vi "get_number_hot_cold_pixels.vi"(8 "error in (no error)":errorcluster, 11 "ColorOverlay in":refnum<class "ColorOverlay.lvclass">) -> (0 "error out":errorcluster, 1 "# hot pixels":i32, 2 "# cold pixels":i32, 3 "ColorOverlay out":refnum<class "ColorOverlay.lvclass">)   [LabVIEW 2010, in "ColorOverlay.lvclass"]
uses:
  ColorOverlay.lvclass
  ColorOverlay.lvclass/ColorOverlay.ctl
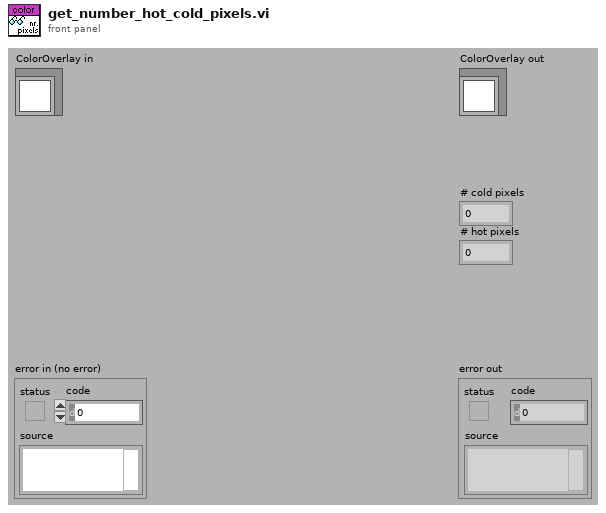
[diagram p1: front panel]
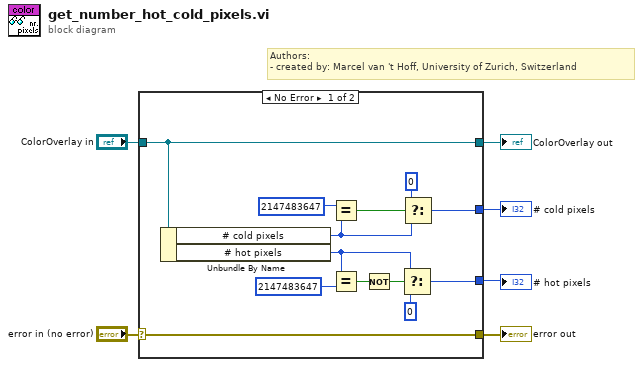
[diagram p0: block diagram]
diagram:
  # "Authors: \n- created by: Marcel van 't Hoff, University of Zurich, Switzerland"
  n1 = case shown="No Error" "error in (no error)" {
    selector: "error in (no error)" -> [w19 w21]
    tunnel: [w19 w21] -> w5
    tunnel: [w18 w20] -> w3
    tunnel: "ColorOverlay in" -> [w18 w20]
    tunnel: [w14 _] -> w2
    tunnel: [w7 _] -> w1
    frame No Error {
      n2 = Unbundle By Name(w18) -> ("# cold pixels"=w15:i32, "# hot pixels"=w8:i32)
      n3 = Equal?(x=2147483647, y=w15) -> (x = y?=w16:bool)
      n4 = Equal?(x=w8, y=2147483647) -> (x = y?=w11:bool)
      n5 = Not(x=w11) -> (.not. x?=w10:bool)
      n6 = Select(t=w8, s=w10, f=0 ("t")) -> (s? t:f=w7:i32)
      n7 = Select(t=0, s=w16, f=w15) -> (s? t:f=w14:i32)
    }
    frame Error {
    }
  }
  "error out" <- w5
  "ColorOverlay out" <- w3
  "# cold pixels" <- w2
  "# hot pixels" <- w1
